vi "Test Report Text Escapes Comma.vi"(11 "Test Case In":refnum<class "Report CSV Content Test.lvclass">) -> (0 "error out":errorcluster, 3 "Test Case Out":refnum<class "Report CSV Content Test.lvclass">)   [LabVIEW 2020, in "Report CSV Content Test.lvclass"]
uses:
  Report CSV Content Test.lvclass
  C:/Program Files (x86)/National Instruments/LabVIEW 2020/vi.lib/Astemes/LUnit/Test Case.lvclass
  source/Configuration/Configuration.lvclass
  <vilib>/Astemes/LUnit/Test Case.lvclass/Test Case.ctl
  <vilib>/Astemes/LUnit/Palette/Fail If.vi
  <vilib>/Astemes/LUnit/Core/LUnit Test Case/Private/Append Pass Result.vi
  <vilib>/Astemes/LUnit/Core/LUnit Test Case/Private/Append Fail Result.vi
  <vilib>/Astemes/LUnit/Core/LUnit Test Case/Private/Run In UI.vi
  <vilib>/Utility/error.llb/Clear Errors.vi
  source/Test Result Handler/TestStand Result Handler.lvclass
  <vilib>/Astemes/LUnit/Palette/Advanced Assertions/LUnit Advanced Assertions.lvlib
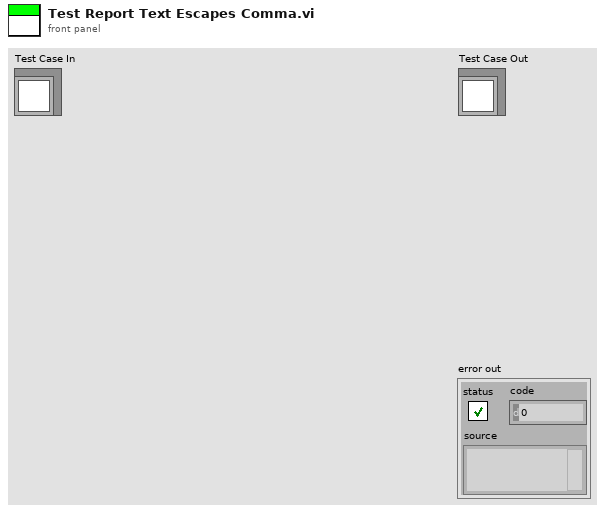
[diagram p1: front panel]
types:
  T1 = typedef "Astemes_CSVReportPlugin.lvlib/TestStand Result Handler.lvclass/TestStand Result.ctl" = cluster{"error in (no error)":errorcluster, "ReportText":string, "TS":cluster{"Index":i32, "BlockLevel":i32, "StartTime":dbl, "Id":i32, "StepType":string, "StepID":string, "StepGroup":string, "StepName":string}, "Status":string}
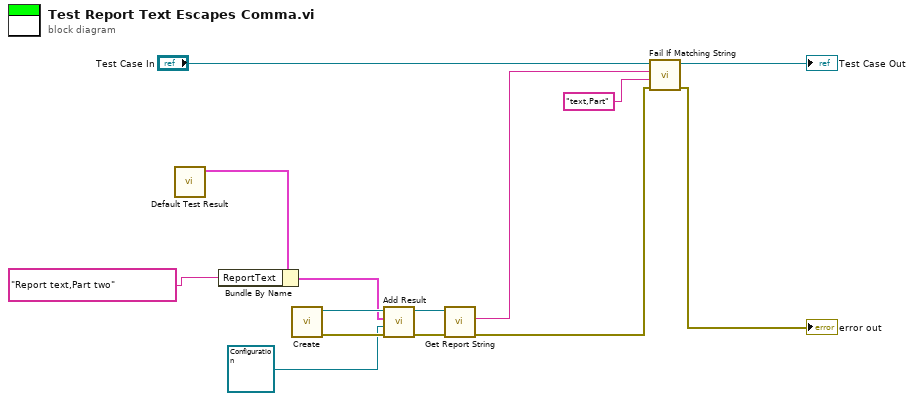
[diagram p0: block diagram]
diagram:
  n1 = call "Default Test Result.vi"() -> ("TestStand Result"=w8:T1)  [unwired: 11 in]
  n2 = Bundle By Name(cluster=w8, "ReportText"="Report text,Part two" ("Status")) -> (w7:T1)
  n3 = call "Create.vi"() -> ("error out"=w11:errorcluster, "Test Result Handler"=w12:refnum<class "TestStand Result Handler.lvclass">)  [unwired: 10 in]
  n4 = call "Add Result.vi"("error in (no error)"=w11, "Sequenc Context"=refnum<class "Configuration.lvclass"> refnum ("Configuration.lvclass"), "TestStand Result"=w7, "TestStand Result Handler In"=w12) -> ("error out"=w9:errorcluster, "TestStand Result Handler Out"=w10:refnum<class "TestStand Result Handler.lvclass">)  [unwired: 6 in]
  n5 = call "Get Report String.vi"("error in (no error)"=w9, "TestStand Result Handler In"=w10) -> ("error out"=w5:errorcluster, "Report Text"=w1:string)  [unwired: 8 in]
  n6 = call <vilib>:"Fail If Matching String.vi"("error in (no error)"=w5, "Regular Expression"="text,Part" ("regular expression"), "String"=w1, "LUnit Test Case In"="Test Case In") -> ("error out"=→"error out":errorcluster, "LUnit Test Case Out"=→"Test Case Out":refnum<class "Report CSV Content Test.lvclass">)  [unwired: 6 in]
